vi "RunInference.vi"(8 "error in (no error)":errorcluster, 11 "ONNX Class in":refnum<class "ONNX Class.lvclass">) -> (0 "error out":errorcluster, 2 "Output Buffer":sgl[](array[numeric]), 3 "ONNX Class out":refnum<class "ONNX Class.lvclass">)   [LabVIEW 2017, in "ONNX Class Library.lvlib" / "ONNX Class.lvclass"]
uses:
  ONNX Class.lvclass
  ONNX Class.lvclass/ONNX Class.ctl
  ONNX Class Library.lvlib
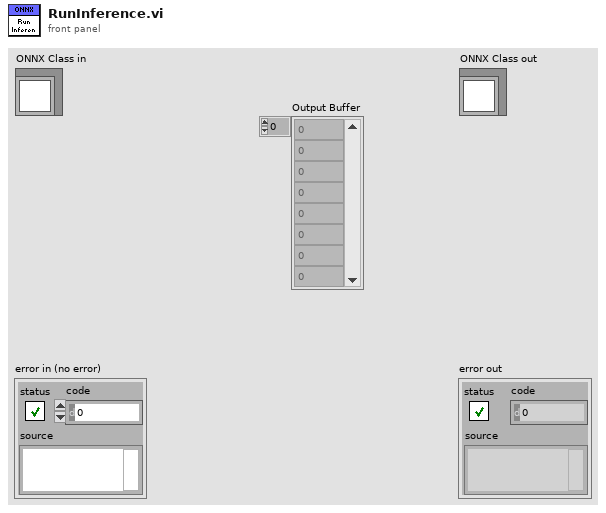
[diagram p1: front panel]
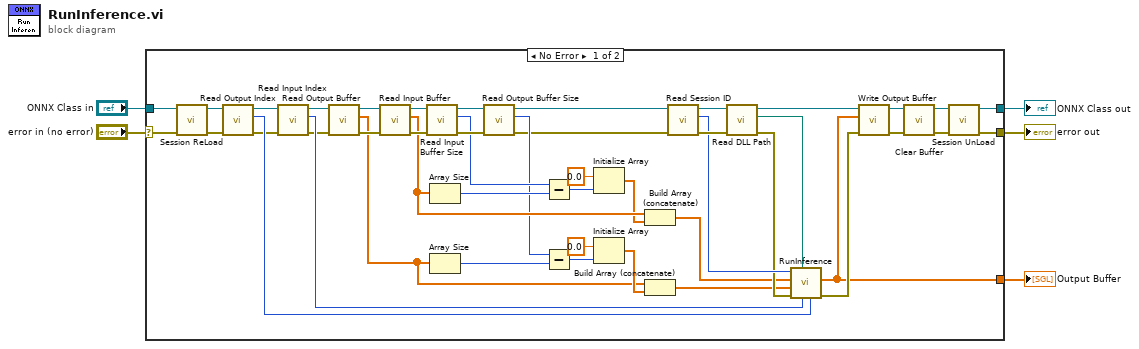
[diagram p0: block diagram]
diagram:
  n1 = case shown="No Error" "error in (no error)" {
    selector: "error in (no error)" -> [w49 w53]
    tunnel: [w41 w53] -> w4
    tunnel: [w42 w52] -> w2
    tunnel: "ONNX Class in" -> [w50 w52]
    tunnel: [w26 _] -> w1
    frame No Error {
      n2 = call-dynamic "Session ReLoad.vi"("error in (no error)"=w49, "ONNX Class in"=w50) -> ("error out"=w35:errorcluster, "ONNX Class out"=w36:refnum<class "ONNX Class.lvclass">)  [unwired: 8 in]
      n3 = call-dynamic "Read Output Index.vi"("error in (no error)"=w35, "ONNX Class in"=w36) -> ("error out"=w33:errorcluster, "Output Index"=w37:i32, "ONNX Class out"=w34:refnum<class "ONNX Class.lvclass">)  [unwired: 7 in]
      n4 = call-dynamic "Read Input Index.vi"("error in (no error)"=w33, "ONNX Class in"=w34) -> ("error out"=w31:errorcluster, "Input Index"=w38:i32, "ONNX Class out"=w32:refnum<class "ONNX Class.lvclass">)  [unwired: 7 in]
      n5 = call-dynamic "Read Output Buffer.vi"("error in (no error)"=w31, "ONNX Class in"=w32) -> ("error out"=w39:errorcluster, "Output Buffer"=w14:sgl[], "ONNX Class out"=w40:refnum<class "ONNX Class.lvclass">)  [unwired: 7 in]
      n6 = call-dynamic "Read Input Buffer.vi"("error in (no error)"=w39, "ONNX Class in"=w40) -> ("error out"=w27:errorcluster, "Input Buffer"=w21:sgl[], "ONNX Class out"=w30:refnum<class "ONNX Class.lvclass">)  [unwired: 7 in]
      n7 = call-dynamic "Read Input Buffer Size.vi"("error in (no error)"=w27, "ONNX Class in"=w30) -> ("error out"=w28:errorcluster, "Input Buffer Size"=w24:i64, "ONNX Class out"=w29:refnum<class "ONNX Class.lvclass">)  [unwired: 7 in]
      n8 = Array Size(array=w21) -> (size(s)=w25:i32)
      n9 = Array Size(array=w14) -> (size(s)=w15:i32)
      n10 = call-dynamic "Read Output Buffer Size.vi"("error in (no error)"=w28, "ONNX Class in"=w29) -> ("error out"=w6:errorcluster, "Output Buffer Size"=w12:i64, "ONNX Class out"=w7:refnum<class "ONNX Class.lvclass">)  [unwired: 7 in]
      n11 = Subtract(x=w24, y=w25) -> (x-y=w23:i64)
      n12 = Subtract(x=w12, y=w15) -> (x-y=w16:i64)
      n13 = Initialize Array(sgl 0.0 ("element"), w23) -> (w20:sgl[])
      n14 = Initialize Array(sgl 0.0 ("element"), w16) -> (w18:sgl[])
      n15 = Build Array (concatenate)(w21, w20) -> (w19:sgl[])
      n16 = Build Array (concatenate)(w14, w18) -> (w13:sgl[])
      n17 = call-dynamic "Read Session ID.vi"("error in (no error)"=w6, "ONNX Class in"=w7) -> ("error out"=w47:errorcluster, "Session ID"=w46:i32, "ONNX Class out"=w48:refnum<class "ONNX Class.lvclass">)  [unwired: 7 in]
      n18 = call-dynamic "Read DLL Path.vi"("error in (no error)"=w47, "ONNX Class in"=w48) -> ("error out"=w45:errorcluster, "DLL Path"=w44:path, "ONNX Class out"=w43:refnum<class "ONNX Class.lvclass">)  [unwired: 7 in]
      n19 = call "RunInference.vi"("Output Index"=w37, "Input Index"=w38, "DLL path"=w44, "error in (no error)"=w45, "Output Buffer"=w13, "Input Buffer"=w19, "session id in"=w46) -> ("error out"=w51:errorcluster, "outputBuffer"=w26:sgl[])  [unwired: 2 in, 1 out]
      n20 = call-dynamic "Write Output Buffer.vi"("error in (no error)"=w51, "Output Buffer"=w26, "ONNX Class in"=w43) -> ("error out"=w10:errorcluster, "ONNX Class out"=w11:refnum<class "ONNX Class.lvclass">)  [unwired: 7 in]
      n21 = call-dynamic "Clear Buffer.vi"("error in (no error)"=w10, "ONNX Class in"=w11) -> ("error out"=w8:errorcluster, "ONNX Class out"=w9:refnum<class "ONNX Class.lvclass">)  [unwired: 8 in]
      n22 = call-dynamic "Session UnLoad.vi"("error in (no error)"=w8, "ONNX Class in"=w9) -> ("error out"=w41:errorcluster, "ONNX Class out"=w42:refnum<class "ONNX Class.lvclass">)  [unwired: 8 in]
    }
    frame Error {
    }
  }
  "error out" <- w4
  "ONNX Class out" <- w2
  "Output Buffer" <- w1
